vi "p2.vi"() -> ()   [LabVIEW 2023, in "d7.lvlib"]
uses:
  d7.lvlib
  <vilib>/regexp/Match Regular Expression.xnode
  AOC/AOC.lvlib
panel:
  out "Answer":u64=1141028
  in  "Example":string="32T3K 765\nT55J5 684\nKK677 28\nKTJJT 220\nQQQJA 483"
  in  "Example":bool=TRUE
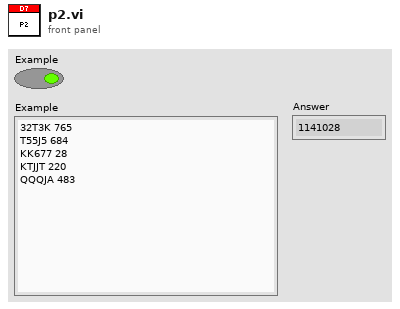
[diagram p1: front panel]
types:
  T1 = cluster{"Cards":i32[], "Type":enum16{"high card", "pair", "two pair", "3 of a kind", "full house", "4 of a kind", "5 of a kind"}, "Bid":u64, "Hand":string}[]
  T2 = cluster{"Cards":i32[], "Type":enum16{"high card", "pair", "two pair", "3 of a kind", "full house", "4 of a kind", "5 of a kind"}, "Bid":u64, "Hand":string}
  T3 = enum16{"high card", "pair", "two pair", "3 of a kind", "full house", "4 of a kind", "5 of a kind"}
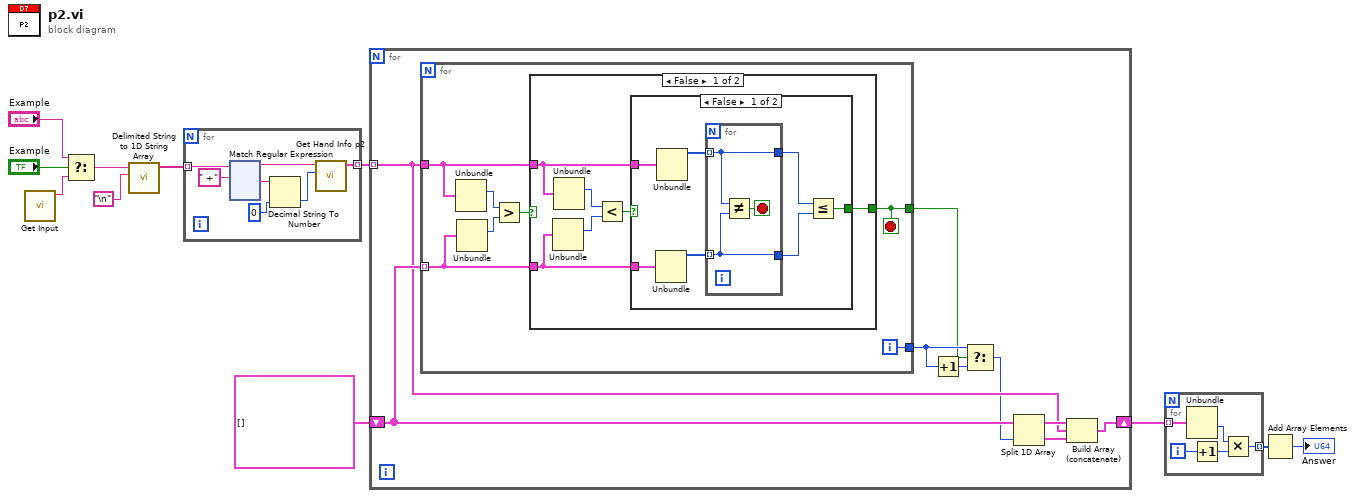
[diagram p0: block diagram]
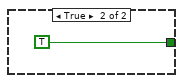
[diagram p2: hidden frame]
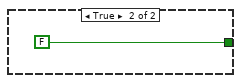
[diagram p3: hidden frame]
diagram:
  n1 = call "Get Input.vi"() -> ("Input"=w11:string)  [unwired: 11 in]
  n2 = Select(t="Example", s="Example", f=w11) -> (s? t:f=w8:string)
  n3 = call <vilib>:"Delimited String to 1D String Array.vi"("delimiter"="\n", "delimited string"=w8) -> ("string array"=w6:string[])  [unwired: 9 in]
  n4 = for {
    tunnel: w6 -> [w18] mode=indexing
    tunnel: [w14] -> w5 mode=indexing
    n5 = xnode "Match Regular Expression"("input string"=w18, "regular expression"=" +") -> ("before match"=w15:string, "after match"=w16:string)  [unwired: 4 in, 3 out]
    n6 = Decimal String To Number(string=w16, default (0L)=u64 0 ("default (0 I32)")) -> (number=w12:u64)  [unwired: 1 in, 1 out]
    n7 = call "Get Hand Info p2.vi"("Bid"=w12, "Hand"=w15) -> ("Hand Info"=w14:T2)  [unwired: 9 in]
  }
  n8 = for {
    tunnel: w5 -> [w141] mode=indexing
    shift-right: [w140] -> w3
    shift-left: T1 [] -> [w144]
    n9 = for {
      tunnel: w144 -> [w148] mode=indexing
      tunnel: w141 -> [w149]
      tunnel: [w150] -> w138
      tunnel: [w145] -> w136
      i -> [w150]
      stop <- w145 stop-if-true
      n10 = Unbundle(w149) -> ("Type"=w147:T3)  [unwired: 3 out]
      n11 = Unbundle(w148) -> ("Type"=w146:T3)  [unwired: 3 out]
      n12 = Greater?(x=w147, y=w146) -> (0:w151:bool)
      n13 = case shown="False" w151 {
        tunnel: [w156 FALSE] -> w145
        tunnel: w149 -> [w153 _]
        tunnel: w148 -> [w152 _]
        frame False {
          n14 = Unbundle(w152) -> ("Type"=w155:T3)  [unwired: 3 out]
          n15 = Unbundle(w153) -> ("Type"=w154:T3)  [unwired: 3 out]
          n16 = Less?(x=w154, y=w155) -> (x < y?=w157:bool)
          n17 = case shown="False" w157 {
            tunnel: [w160 TRUE] -> w156
            tunnel: w153 -> [w164 _]
            tunnel: w152 -> [w163 _]
            frame False {
              n18 = Unbundle(w163) -> ("Cards"=w161:i32[])  [unwired: 3 out]
              n19 = Unbundle(w164) -> ("Cards"=w162:i32[])  [unwired: 3 out]
              n20 = for {
                tunnel: w162 -> [w167] mode=indexing
                tunnel: w161 -> [w166] mode=indexing
                tunnel: [w167] -> w159
                tunnel: [w166] -> w158
                stop <- w165 stop-if-true
                n21 = Not Equal?(x=w167, y=w166) -> (x != y?=w165:bool)
              }
              n22 = Less Or Equal?(x=w159, y=w158) -> (x <= y?=w160:bool)
            }
            frame True {
            }
          }
        }
        frame True {
        }
      }
    }
    n23 = Increment(x=w138) -> (x+1=w137:i32)
    n24 = Select(t=w138, s=w136, f=w137) -> (s? t:f=w139:i32)
    n25 = Split 1D Array(array=w144, index=w139) -> (first subarray=w143:T1, second subarray=w142:T1)
    n26 = Build Array (concatenate)(w143, w141, w142) -> (w140:T1)
  }
  n27 = for {
    tunnel: w3 -> [w174] mode=indexing
    tunnel: [w170] -> w2 mode=indexing
    i -> [w173]
    n28 = Unbundle(w174) -> ("Bid"=w172:u64)  [unwired: 3 out]
    n29 = Increment(x=w173) -> (x+1=w171:i32)
    n30 = Multiply(x=w172, y=w171) -> (x*y=w170:u64)
  }
  n31 = Add Array Elements(numeric array=w2) -> (sum=→"Answer":u64)
